vi "input_channel.vi"() -> ()   [LabVIEW 2017]
uses:
  input_channel.ctl
panel:
  in  "Analog Input Channels":T1[](array[typedef]) {"TC Type" items=["J"=10072, "K"=10073, "N"=10077, "R"=10082, "S"=10085, "T"=10086, "B"=10047, "E"=10055]; "Output Offset" format="%0.5f"; "Gain(Slope)" format="%0.5f"; "Input Offset" format="%0.5f"; "Maximum Value" format="%0.5f"; "Minimum Value" format="%0.5f"; "Terminal Configuration" items=["Default"=-1, "RSE"=10083, "NRSE"=10078, "Differential"=10106, "Pseudodifferential"=12529]; "Signal Type" items=["Voltage", "Current", "Temperature"]; "Sensor Type" items=["Absolute Pressure", "Gauge Pressure", "Differential Pressure", "Temperature", "Mass Flow Rate", "Density", "Other"]}
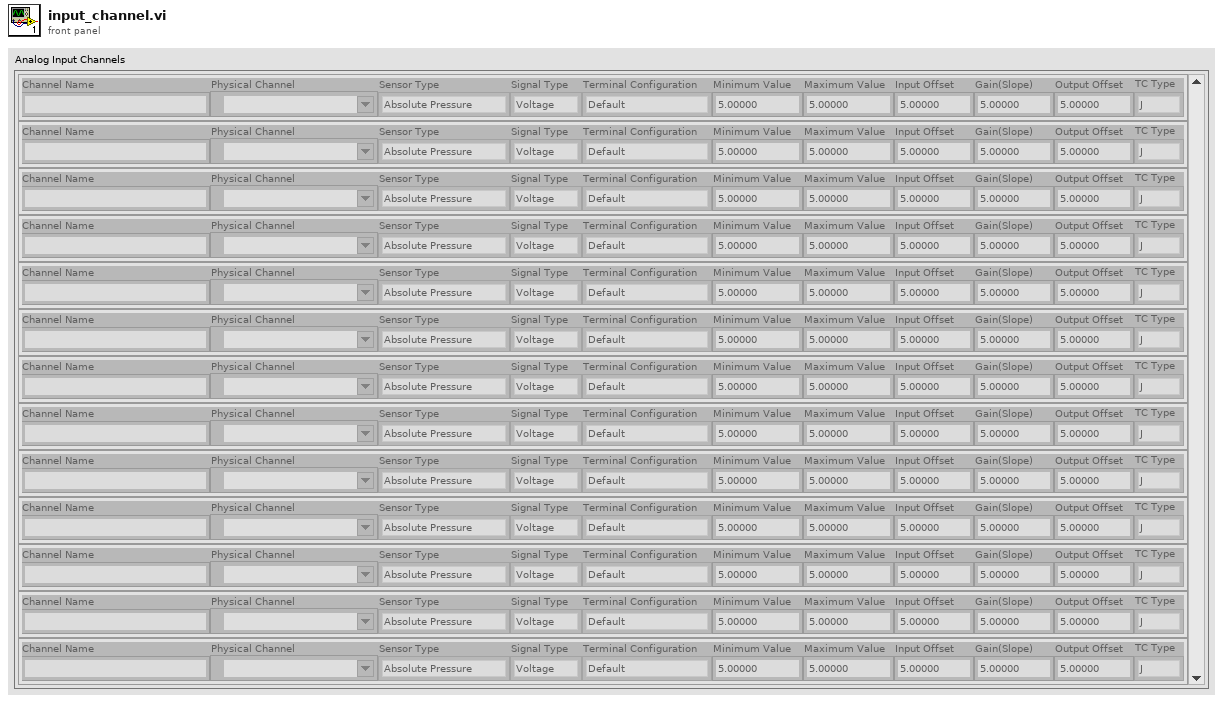
[diagram p1: front panel]
types:
  T1 = typedef "input_channel.ctl" = cluster{"Channel Name":string, "Sensor Type":i32, "Signal Type":i32, "Terminal Configuration":i32, "Physical Channel":tag, "Minimum Value":dbl, "Maximum Value":dbl, "Input Offset":dbl, "Gain(Slope)":dbl, "Output Offset":dbl, "TC Type":i32}
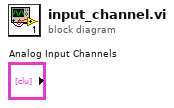
[diagram p0: block diagram]
diagram:
